vi "Day 15 - Beacon Exclusion Zone.vi"() -> ()   [LabVIEW 2020, in "AoC 2022.lvlib"]
uses:
  AoC 2022.lvlib
panel:
  out "Area Centroids":cluster{"Centroid X":dbl, "Centroid Y":dbl}[](array[cluster])
  out "Area That Can Contain Beacons":cluster{cluster{"X":dbl, "Y":dbl}[]}[](graph)
  out "Puzzle Part-2 Answer":dbl[](array[numeric]) format="%#_15f"
  in  "F:Part 1 | T:Part 2":bool
  in  "Boundary":T1={"X Max"=4000000, "X Min"=0, "Y Max"=4000000, "Y Min"=0}
  in  "Y Row to Check":i32=2000000
  in  "Puzzle Input":string="Sensor at x=2, y=18: closest beacon is at x=-2, y=15\nSensor at x=9, y=16: closest beacon is at x=10, y=16\nSensor at x=13, y=2: closest beacon is at x=15, y=3\nSensor at x=12, y=14: closest beacon is at x=10, y=16\nSensor at x=10, y=20: closest beacon is at x=10, y=16\nSensor at x=14, y=17: closest beacon is at x=10, y=16\nSensor at x=8, y=7: closest beacon is at x=2, y=10\nSensor at x=2, y=0: closest beacon is at x=2, y=10\nSensor at x=0, y=11: closest beacon is at x=2, y=10\nSensor at x=20, y=14: closest beacon is at x=25, y=17\nSensor at x=17, y=20: closest beacon is at x=21, y=22\nSensor at x=16, y=7: closest beacon is at x=15, y=3\nSensor at x=14, y=3: closest beacon is at x=15, y=3\nSensor at x=20, y=1: closest beacon is at x=15, y=3"
  out "Puzzle Answer":string
  # "Press Ctrl+M & Enter the Puzzle Input and run the VI"
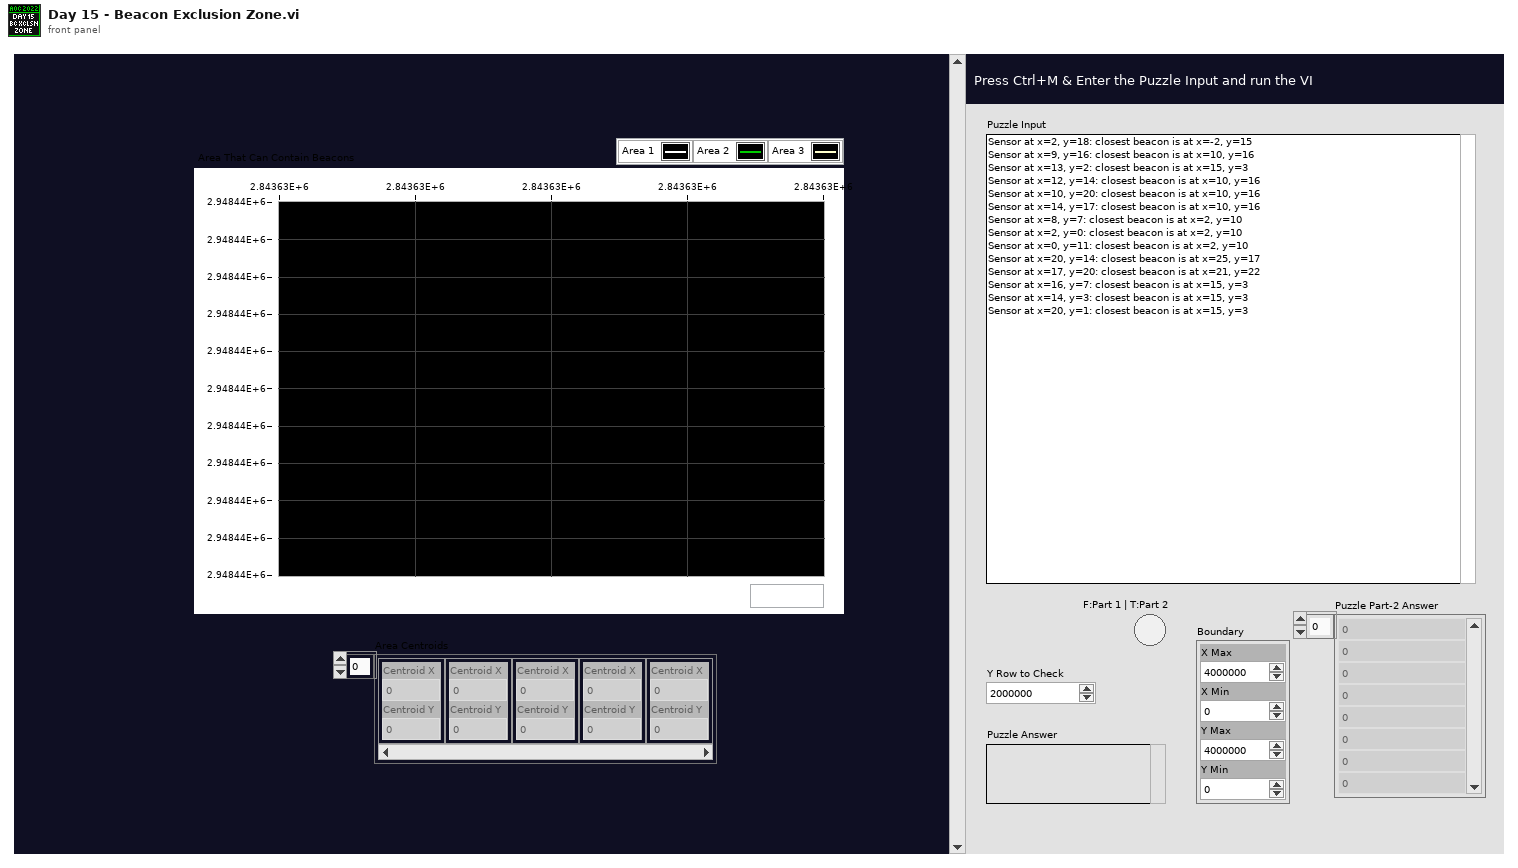
[diagram p1: front panel]
types:
  T1 = cluster{"X Max":i32, "X Min":i32, "Y Max":i32, "Y Min":i32}
  T2 = typedef "AoC 2022.lvlib/Location.ctl" = cluster{"X":i32, "Y":i32}
  T3 = typedef "AoC 2022.lvlib/Sensor Info.ctl" = cluster{"Beacon":T2, "Distance to Beacon":dbl, "Coverage Area":T4}
  T4 = typedef "AoC 2022.lvlib/Coverage Area.ctl" = cluster{"X":dbl[], "Y":dbl[]}
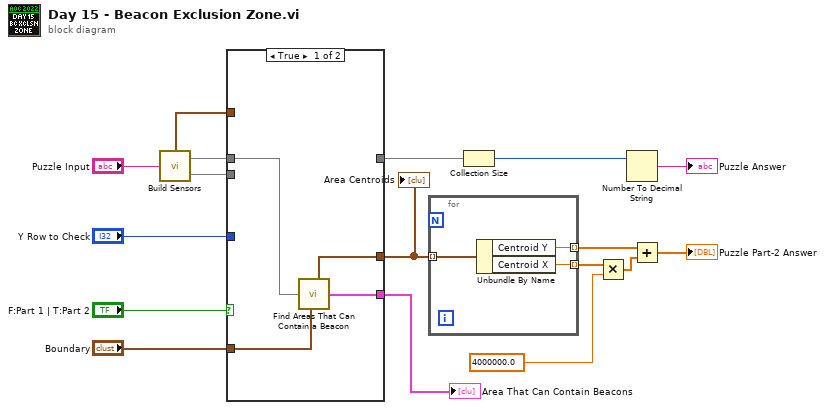
[diagram p0: block diagram]
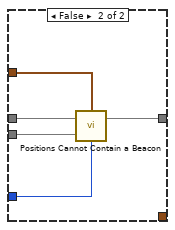
[diagram p2: hidden frame]
diagram:
  n1 = call "Build Sensors.vi"("Puzzle Input"="Puzzle Input") -> ("Boundary"=w15:T1, "Sensors"=w11:map{T2, T3}, "Beacons"=w10:set{T2})
  n2 = case shown="True" "F:Part 1 | T:Part 2" {
    tunnel: w15 -> [_ w26]
    tunnel: [_ w25] -> w14
    tunnel: "Y Row to Check" -> [_ w24]
    tunnel: w11 -> [w21 w23]
    tunnel: w10 -> [_ w22]
    tunnel: "Boundary" -> [w20 _]
    tunnel: [w19 _] -> w3
    tunnel: [w18 _] -> w1
    frame True {
      n3 = call "Find Areas That Can Contain a Beacon.vi"("Sensors"=w21, "Boundary"=w20) -> ("Area Centroids"=w19:cluster{"Centroid X":dbl, "Centroid Y":dbl}[], "Area That Can Contain Beacons"=w18:cluster{cluster{"X":dbl, "Y":dbl}[]}[])
    }
    frame False {
      n4 = call "Positions Cannot Contain a Beacon.vi"("Beacons"=w22, "Y Row to Check"=w24, "Sensors"=w23, "Boundary"=w26) -> ("Positions Cannot Contain a Beacon"=w25:set{T2})  [unwired: 1 in]
    }
  }
  "Area That Can Contain Beacons" <- w1
  "Area Centroids" <- w3
  n5 = for {
    tunnel: [w29] -> w8 mode=indexing
    tunnel: [w28] -> w5 mode=indexing
    tunnel: w3 -> [w27] mode=indexing
    n6 = Unbundle By Name(w27) -> ("Centroid Y"=w28:dbl, "Centroid X"=w29:dbl)
  }
  n7 = Collection Size(1:w14) -> (0:w12:i32)
  n8 = Multiply(x=w8, y=4000000.0) -> (x*y=w6:dbl[])
  n9 = Number To Decimal String(number=w12) -> (decimal integer string=→"Puzzle Answer":string)  [unwired: 1 in]
  n10 = Add(x=w5, y=w6) -> (x+y=→"Puzzle Part-2 Answer":dbl[])
